vi "Center Map on.vi"(8 "Error In":errorcluster, 9 "lng":dbl, 11 "lat":dbl) -> (0 "error out":errorcluster)   [LabVIEW 2014]
uses:
  C:/Robotic Systems/Products/Surveyor/Software/Ground Station/Data/Mapping DLL/GMap.NET.Core.dll
  Data/Mapping DLL/GMap.NET.Core.dll
  C:/Robotic Systems/Products/Surveyor/Software/Ground Station/Data/Mapping DLL/GMap.NET.WindowsForms.dll
  Data/Mapping DLL/GMap.NET.WindowsForms.dll
  Reference/SubVI/GMap DLL Refernce.vi
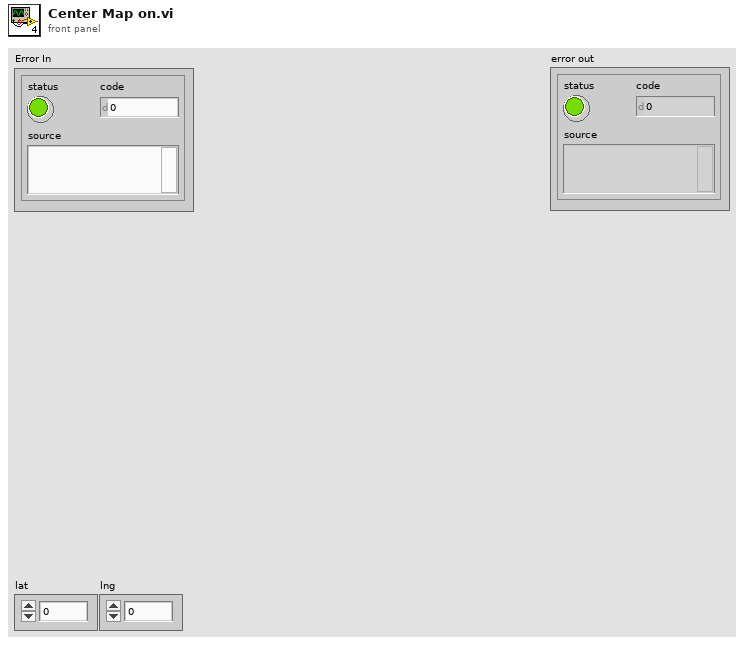
[diagram p1: front panel]
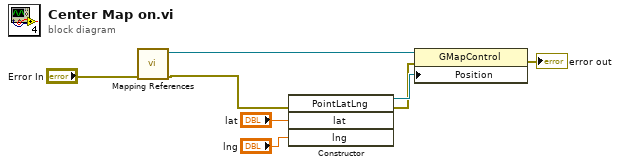
[diagram p0: block diagram]
diagram:
  n1 = call-poly "Mapping References.vi"("Error In"="Error In") -> ("Error Out"=w4:errorcluster, "GMap DLL Reference"=w5:refnum<k24>)  [unwired: 9 in]
  n2 = constructor class="PointLatLng"(error in=w4, "lat"="lat", "lng"="lng") -> (reference out=w8:refnum<k24>, error out=w3:errorcluster)  [unwired: 2 in, 3 out]
  n3 = property class="GMapControl"(reference=w5, error in=w3, "Position"=w8) -> (error out=→"error out":errorcluster)  [unwired: 1 out]
